vi "Práctica01_Ejercicio3_2.vi"() -> ()   [LabVIEW 2020]
uses:
  <vilib>/numeric/Random Number (Range) DBL.vi
panel:
  out "Numeric":dbl
  out "Valor máximo Señal 2":dbl
  out "Valor máximo Señal 1":dbl
  out "GRÁFICA DE SEÑALES":dynamicdata(graph)
  out "Señal 2":dbl[](array[numeric])
  out "Señal 1":dbl[](array[numeric])
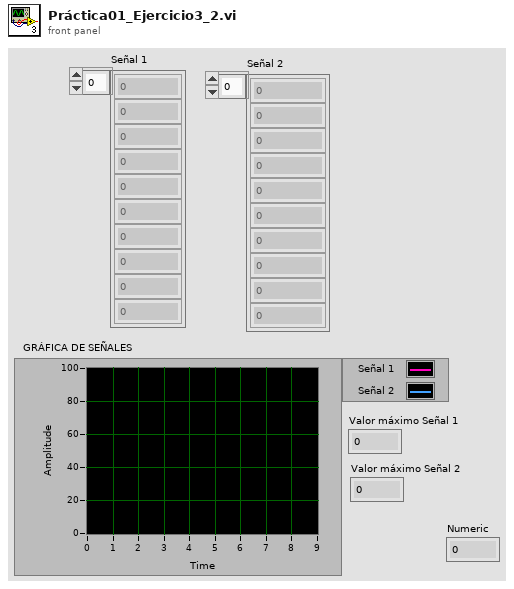
[diagram p1: front panel]
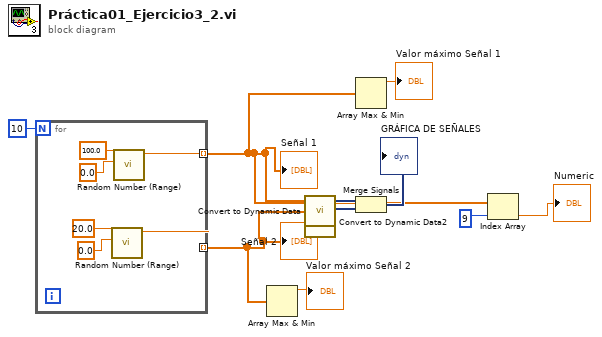
[diagram p0: block diagram]
diagram:
  n1 = for {
    N: 10 -> [_]
    tunnel: [w14] -> w3 mode=indexing
    tunnel: [w11] -> w5 mode=indexing
    n2 = call-poly <vilib>:"Random Number (Range).vi"("lower bound (0)"=0.0, "upper bound (100)"=20.0) -> ("number"=w11:dbl)  [unwired: 9 in]
    n3 = call-poly <vilib>:"Random Number (Range).vi"("lower bound (0)"=0.0, "upper bound (100)"=100.0) -> ("number"=w14:dbl)  [unwired: 9 in]
  }
  "Señal 1" <- w3
  "Señal 2" <- w5
  n4 = Array Max & Min(array=w5) -> (max value=→"Valor máximo Señal 2":dbl)  [unwired: 3 out]
  n5 = call "Convert to Dynamic Data"("Array"=w3) -> ("Dynamic Data Type"=w9:dynamicdata)  [unwired: 3 in]
  n6 = call "Convert to Dynamic Data2"("Array"=w5) -> ("Dynamic Data Type"=w8:dynamicdata)  [unwired: 3 in]
  n7 = Array Max & Min(array=w3) -> (max value=→"Valor máximo Señal 1":dbl)  [unwired: 3 out]
  n8 = Merge Signals "Merge Signals"(w9, w8) -> (→"GRÁFICA DE SEÑALES":dynamicdata)
  n9 = Index Array(array=w3, index=9) -> (element=→"Numeric":dbl)
